vi "Set Home Transform T0.vi"(8 "error in (no error)":errorcluster, 10 "T0 Transform":T1, 11 "Robot Arm in":refnum<class "Robot Arm.lvclass">) -> (0 "error out":errorcluster, 3 "Robot Arm out":refnum<class "Robot Arm.lvclass">)   [LabVIEW 2013, in "Robot Arm.lvclass"]
uses:
  Robot Arm.lvclass
  <vilib>/Analysis/Matrix/Datatypes/RealMatrix.ctl
  Robot Arm.lvclass/Robot Arm.ctl
  <vilib>/Analysis/Matrix/NI_Matrix.lvlib
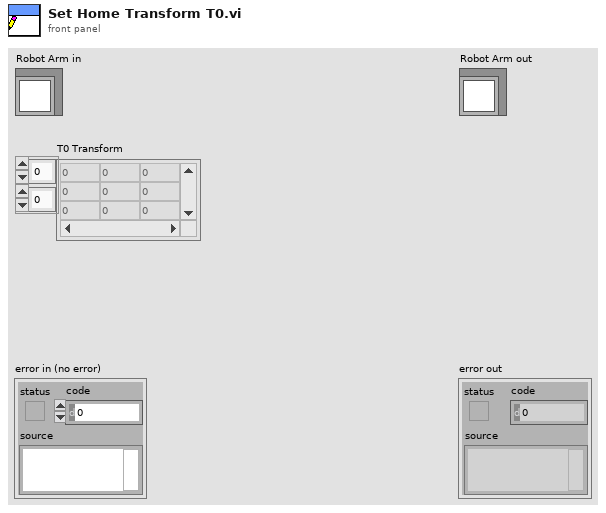
[diagram p1: front panel]
types:
  T1 = typedef "NI_Matrix.lvlib/RealMatrix.ctl" = dbl[][]
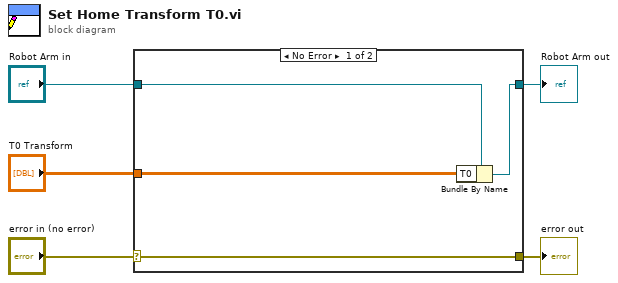
[diagram p0: block diagram]
diagram:
  n1 = case shown="No Error" "error in (no error)" {
    selector: "error in (no error)" -> [w9 w10]
    tunnel: [w9 w10] -> w4
    tunnel: [w7 w11] -> w2
    tunnel: "Robot Arm in" -> [w8 w11]
    tunnel: "T0 Transform" -> [w6 _]
    frame No Error {
      n2 = Bundle By Name(cluster=w8, "T0"=w6) -> (w7:refnum<class "Robot Arm.lvclass">)
    }
    frame Error {
    }
  }
  "error out" <- w4
  "Robot Arm out" <- w2
